vi "AlliGator All ROIs Decay Fit.vi"(8 "error in (no error)":errorcluster, 10 "Lifetime Graph":refnum<vi>, 11 "AlliGator Internal Variables DVR":refnum<data-value>) -> (0 "error out":errorcluster, 1 "Message":string, 3 "AlliGator Internal Variables DVR":refnum<data-value>)   [LabVIEW 2021, in "AlliGator Decay Analysis.lvlib" / "AlliGator Decay Fit.lvlib"]
doc: "Fits all ROI decays with the selected model, using a common IRF for all ROIs."
uses:
  AlliGator Decay Fit.lvlib
  AlliGator Variables List.ctl
  AlliGator Globals, Variables & Constants.lvlib
  Image/Named ROI Description.ctl
  Image/Image.lvlib
  AlliGator Decay Processing.lvlib
  AlliGator Source Image.lvlib
  Strings/Strings.lvlib
  Time/Time.lvlib
  Graphs/XY Graph/XY Graph Add-Ons.lvlib
  AlliGator Settings.lvlib
  AlliGator Settings List.ctl
  Graphs/XY Graph/XY Graph Selected Plot Info+Flag.ctl
  <vilib>/Utility/miscctls.llb/LVPoint32TypeDef.ctl
  Graphs/XY Graph/XY Graph Refnum.ctl
  AlliGator Decay Preprocessing.lvlib
  AlliGator Abort.vi
  Fits/Fits.lvlib
  Variant/Variant to Data/Variant to Data.lvlib
  Variant/Variant to Data/Variant to Boolean.vi
  <vilib>/ErrorRing/Error Ring.xnode
  Notebook/Notebook.lvlib
  Rich Text Box/Rich Text Box.lvlib
  <vilib>/vision/Image Controls.llb/IMAQ Image.ctl
  <vilib>/Utility/error.llb/Error Cluster From Error Code.vi
  GUI/GUI.lvlib
  Fits/IRF(X)PSED/Decay Fit Parameters & Derived Quantities List.ctl
  Utilities/Utilities.lvlib
  Error/Error.lvlib
  Variant/Variant to Data/Variant to U16.vi
  AlliGator Decay Fit Parameter Map.lvlib
  Phasor/Phasor Reference Series.ctl
  Phasor/Phasor.lvlib
  Phasor/Phasor (g, s).ctl
  Phasor/Calibration Phasor (m, phi).ctl
  AlliGator Data Series Type.ctl
  AlliGator Files.lvlib
  AlliGator Internal Variables v2.ctl
  AlliGator Internal Variables.lvlib
  AlliGator Decay Metadata v3.ctl
  AlliGator Phasor Graph.lvlib
  AlliGator Raw Phasor Plot Data v4.ctl
  AlliGator Baseline Subtraction Method.ctl
  AlliGator Decay Background Subtraction Info.ctl
  Graphs/XY Graph/XY Graph Plot Shift Method.ctl
  Graphs/XY Graph/XY Graph Plot Shift Parameters.ctl
  AlliGator Decay Extrapolation Parameters.ctl
  AlliGator FLI Dataset Type.ctl
  Phasor/Phasor Harmonic Data.ctl
  AlliGator Phasor Multi-Harmonic Data.ctl
  AlliGator Phasor Plot.lvlib
  AlliGator Displayed Image.ctl
  Fits/IRF(X)PSED/Decay Fit Parameters In List.ctl
  AlliGator Decay Fit Parameter Constraints 2.ctl
  Fits/Decay Convolution/Decay Model.ctl
  Fits/Residual Type.ctl
  Fits/Fit Calculation Method.ctl
  Fits/Non-linear Fitting Algorithm.ctl
  AlliGator Decay Fit Options & Parameters v2.ctl
  Fits/IRF(X)PSED/Fit Weights Type.ctl
  AlliGator Gate Image Set.ctl
  AlliGator Gate Arithmetic.ctl
  AlliGator Dataset Channel.ctl
  AlliGator Dual-Channel Datasets.lvlib
  AlliGator Decay Preprocessing Parameters.ctl
  Phasor/Phasor Standard Deviation Options.ctl
  Phasor/Phasor Calibration Map v2.ctl
  Fits/Non-linear Fitting Method v2.ctl
  Fits/IRF(X)PSED/Decay Fit Options v2.ctl
  Fits/IRF(X)PSED/MLE Baseline Offset Type.ctl
  AlliGator Parameter Maps Data.ctl
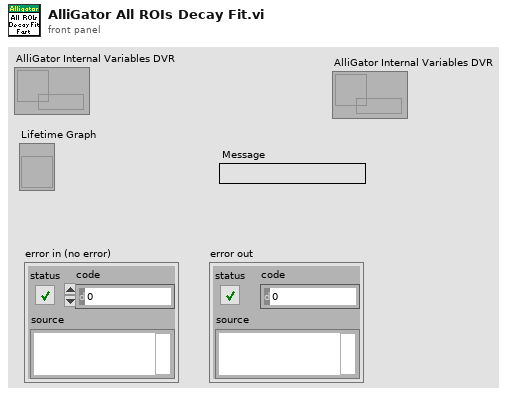
[diagram p1: front panel]
types:
  T1 = typedef "AlliGator Decay Analysis.lvlib/AlliGator Decay Fit.lvlib/AlliGator Decay Fit Output Options.ctl" = cluster{"Fit Model":T2, "Decay Fit Parameter Array":T3[]}
  T2 = typedef "Fits.lvlib/Decay Model.ctl" = enum16{"1-Exponential", "2-Exponentials"}
  T3 = typedef "Fits.lvlib/Decay Fit Parameters & Derived Quantities List.ctl" = enum16{"Offset", "Baseline", "A_1", "tau_1", "A_2", "tau_2", "<tau>_a", "f1_a", "f2_a", "<tau>_i", "f1_i", "f2_i", "-", "R^2", "Chi^2"}
  T4 = typedef "AlliGator Globals, Variables & Constants.lvlib/AlliGator Variables List.ctl" = enum16{"---- GUI ----", "GUI:Initialization Status", "GUI:State Indicators Refnum", "GUI:Original AlliGator Menu Items", "GUI:Current Action Loop State", "GUI:Script in progress", "GUI:Playback", "GUI:Loop Playback", "GUI:Search ROI Used", "GUI:Search ROI", "Decay Graph Max Legend Size", "Intensity Graph Max Legend Size", "Decay Statistics Graph Max Legend Size", "Phasor Graph Max Legend Size", "Phasor Ratio Graph Max Legend Size", "Lifetime Graph Max Legend Size", "---- Files ----", "Files:Export Dataset Frames as Individual Files", "Files:Show Batch Export Help Balloons", "Files:Frames in Dataset", "Files:ptu File Frame Start Indices", "Files:Current Frame in Dataset", "Files:Current Frame Timestamp", "Files:Dataset Loaded", "Files:Dataset Metadata", "Files:Dataset Channel", "Files:Dataset Data Description", "Files:Background Dataset Metadata", "Files:Background Dataset Channel", "Files:Background Dataset Data Description", "Files:Background File Subtraction", "Files:Background File Path", "Files:Background File Pile-up Correction", "Files:Background File Pixel Well Capacity", "Files:Background File Scaling Factor", "Files:Current Dataset Load Settings", "Files:Dataset Path", "Files:ICCD-specific Information", "Files:Macrotime Gate Separation", "------ Python Plugins ------", "Python Plugins:Information", "Python Plugins:Python Session", "Python Plugins:Valid Python Session?", "---- Source Image ----", "Source Image:ROIs", "Source Image:Current ROI", "Source Image:ROI Event Refnum", "X_Source Image Display Range", "X_Source Image Palette Information", "X_Type of Displayed Image", "X_Time Gate Slider", "Source Image:Palette List", "Source Image:Scale", "Source Image:ROI Overlay Color", "Source Image:Overlay to Erase", "Source Image:Is Displayed Image Accumulated", "Source Image:White Light Image Modified", "Source Image:Mask Image Modified", "---- Image Profile Window ----", "Image Profile:Overlay ROI in Source Image", "Image Profile:Window Event Refnum", "Image Profile:IntensityType", "Image Profile:Intensity Average Type", "Image Profile:Intensity-weighted SDV", "Image Profile:Box Profile Type", "Image Profile:Window Open", "Image Profile:Plotted Fit Parameter", "------ Phasor Graph -------", "Phasor Graph:Show Line", "---- Phasor Plot ---", "Phasor Plot:Parameters Changed", "Phasor Plot:FLI Dataset Modified since last Calculation", "Phasor Harmonics Data", "Selected Phasor Harmonics", "Phasor Harmonic Manager Event Refnum", "Phasor Plot:ROIs", "Phasor Plot:Current ROI", "Phasor Plot:ROI Event Refnum", "Phasor Plot:Image Reference Points", "Phasor Plot:Computed", "Phasor Plot:Palette Information", "Phasor Plot:Palette List", "Phasor Plot:Phasor Ratio Palette Information", "Phasor Plot:Phasor Ratio Palette List", "Phasor Plot:Image Scale", "Phasor Plot:Image Overlay to Erase", "Phasor Plot:Image Elements to Update", "Phasor Plot:Current Calculation Parameters", "Phasor Plot:Current Calibration Options", "Phasor Plot:Reset Cumulated Phasor Plot", "Phasor Plot:Reference 1", "Phasor Plot:Lifetime Reference 1", "Phasor Plot:Reference 1 Frequency", "Phasor Plot:Reference 2", "Phasor Plot:Lifetime Reference 2", "Phasor Plot:Reference 2 Frequency", "---- Decay Analysis ----", "Number of Selected Decays to Fit", "LS Fit Results", "LAR Fit Results", "BS Fit Results", "Last Decay Max - Min", "Best Fit Parameters", "Best Fit Parameter Names", "Actual Size X", "Actual Size Y", "Binning X", "Binning Y", "Actual # Gates", "Dataset Number", "Gates to...", "Gates Skipped", "Gates to keep", "Gate Step", "Gate Separation", "Reversed Gates", "Pile-up Correction", "Pixel Well Capacity", "Background Subtracted", "Background Subtraction Method", "Background Definition Range", "Background File (deprecated)", "Number of Dataset Accumulated", "Array of Accumulated Dataset Paths", "Do Averaged Datasets", "Destination File Path", "Process Plot Target", "Use 1/D as Phasor Frequency", "---- Decay Fit Parameter Map -----", "Decay Fit Parameter Map:Palette Information", "Decay Fit Parameter Map:Palette List", "------- Local Decay Window ---------", "Local Decay Graph Window:Event Refnum", "Local Decay Graph Window:Use normalized IRF for convolution", "----- Miscellaneous ----", "Misc:Skippable Dialog Windows Status"}
  T5 = typedef "IMAQ Image.ctl" = refnum<image>
  T6 = typedef "AlliGator Settings.lvlib/AlliGator Settings List.ctl" = enum16{"GUI:Visible Settings Tab", "GUI:Last Run Version", "Source Image:Use Image Histogram for Contrast", "Source Image:Low Count Pixels Rejection Options", "Source Image:High Count Pixels Rejection Options", "Source Image:Use Image Brightness", "Source Image:Blend Overlay with Image Background", "Source Image:Use Fixed ROI Diameter", "Source Image:ROI Diameter", "Source Image:ROI Center Color", "Source Image:Peak Threshold", "Source Image:Intensity Threshold", "Source Image:Image Binning Options", "Source Image:Image Smoothing Options", "Source Image:Image Histogram Active", "Source Image:Invert Binary Mask", "Source Image:Hot Pixel Removal", "Source Image:Overlay Analyzed ROI Center", "Source Image:Auto-Adjust Contrast", "Source Image:Histogram Lower Percentile", "Source Image:Histogram Upper Percentile", "Source Image:Save Source Image", "Source Image:Scale Bar Options", "Source Image:Image Resolution (Pixel Size)", "Source Image:Flatfield Correction", "Source Image:Show Dead Left Columns Correction", "Source Image:Dead Left Columns Correction", "Source Image:Image Pre-Processing Operations Order", "Data Information:Gate Width", "Data Information:Nanotime Gate Separation", "Data Information:Macrotime Gate Separation", "Data Information:Gate Step", "Data Information:# Gates", "Data Information:Gate Image Exposure", "Data Information:Gate Image Integration", "Data Information:Gates to Skip", "Data Information:Gates to Keep", "Data Information:Define Gates to", "Data Information:Channel Name", "Data Information:Available Channel Names", "Data Information:Channel Arithmetic", "Data Information:Background File Subtraction", "Data Information:Background File", "Data Information:Background Scaling Factor", "Data Information:Background Pile-up Correction", "Data Information:Background Pixel Well Capacity", "Data Information:Laser Period", "Data Information:SYNC Period", "Data Information:Pile-up Correction", "Data Information:Pixel Well Capacity", "Data Information:Dataset Scaling Factor", "Fluorescence Decay_Decay Pre-Processing:Reverse Gates", "Fluorescence Decay_Decay Pre-Processing:Verbose Decay Pre-Processing", "Fluorescence Decay_Decay Pre-Processing:Use Decay Pre-Processing", "Fluorescence Decay_Decay Pre-Processing:Background Subtraction", "Fluorescence Decay_Decay Pre-Processing:Background Definition Range", "Fluorescence Decay_Decay Pre-Processing:Baseline Subtraction Method", "Fluorescence Decay_Decay Pre-Processing:Decay Pre-Processing Operations Order", "Fluorescence Decay_Decay Pre-Processing:Smoothing Parameter", "Fluorescence Decay_Decay Pre-Processing:Shift Decay", "Fluorescence Decay_Decay Pre-Processing:Decay Shift Parameters", "Fluorescence Decay_Decay Pre-Processing:Fold Decay", "Fluorescence Decay_Decay Pre-Processing:# Folds", "Fluorescence Decay_Decay Pre-Processing:1-Normalize Decay", "Fluorescence Decay_Decay Pre-Processing:[0-1]-Normalize Decay", "Fluorescence Decay_Decay Pre-Processing:Smoothen Decay", "Fluorescence Decay_Decay Pre-Processing:Extrapolate Decay", "Fluorescence Decay_Decay Pre-Processing:Use Periodicity", "Fluorescence Decay_Decay Pre-Processing:Use Cursors", "Fluorescence Decay_Decay Pre-Processing:Tail Fraction", "Fluorescence Decay_Decay Pre-Processing:Head Fraction", "Fluorescence Decay_Decay Pre-Processing:Additional Points", "Fluorescence Decay_Decay Pre-Processing:Straighten Decay", "Fluorescence Decay_Decay Pre-Processing:Constant Background", "Fluorescence Decay_Decay Pre-Processing:Pixel-Normalize Decay", "Fluorescence Decay_Advanced Analysis:Extract IRF instead of Decay", "Fluorescence Decay_Advanced Analysis:IRF Extraction Options", "Fluorescence Decay_Advanced Analysis:IRF Optimization Options", "Fluorescence Decay_Advanced Analysis:Square Pulse Options", "Fluorescence Decay_Advanced Analysis:IRF Order", "Fluorescence Decay_Advanced Analysis:IRF Time Constants", "Fluorescence Decay_Advanced Analysis:Wavelet Analysis Options", "Fluorescence Decay_Advanced Analysis:Average Lifetime Options", "Fluorescence Decay_Fit Options:Fit Options", "Fluorescence Decay_Fit Options:Use Legacy Fitting Approach", "Fluorescence Decay_Fit Options:Use Data Information Laser Period", "Fluorescence Decay_Fit Parameters:Displayed Fit Parameters", "Fluorescence Decay_Fit Parameters:Fit Parameter Constraints", "Fluorescence Decay_Fit Parameters:Export Tabulated Results", "Fluorescence Decay_Fit Parameters:MLE Baseline Offset Type", "Fluorescence Decay_Fit Parameters:MLE Baseline Offset", "Fluorescence Decay_Fit Parameters:Guess Parameter Names", "Fluorescence Decay_Fit Parameters:Guess Parameter Values", "Fluorescence Decay_Fit Parameters:Guess Parameters Options", "Fluorescence Decay_Styles:Show Last Decay Only", "Fluorescence Decay_Styles:Decay Graph Color Array", "Fluorescence Decay:Decay Graph Active", "Fluorescence Decay Statistics:Min Peak Value", "Fluorescence Decay Statistics:Reject Low Decay Peak Pixels", "Fluorescence Decay Statistics:Reject High Decay Peak Pixels", "Fluorescence Decay Statistics:Max Peak Value", "Time Traces:Use File Timestamp", "Time Traces:Time Step", "Time Traces:Use Intensity Correction File", "Time Traces:Intensity Correction File", "Phasor Plot:Phasor Plot Smoothing Options", "Phasor Plot:Phasor Plot Size", "Phasor Plot:Phasor Plot Graphics Options", "Phasor Plot:Cumulative Phasor Plot", "Phasor Plot:Use Phasor Brightness", "Phasor Plot:Blend Overlay with Phasor Background", "Phasor Plot:Save Phasor Plot", "Phasor Plot:Show References", "Phasor Plot:Phasor Ratio Decay Range", "Phasor Plot:Exponential Fading", "Phasor Plot:Phasor Ratio Reference Colors", "Phasor Plot:Reference Radius", "Phasor Plot:Show Color Map Vertices", "Phasor Plot:Phasor Plot Active", "Phasor Plot:Phasor Ratio Color Map Type", "Phasor Plot:Phasor Ratio Color Map", "Phasor Plot:Phasor Ratio Display Range", "Phasor Plot:Selected Image ROI(s)", "Phasor Plot:All Image ROIs", "Phasor Plot:Selected Phasor Plot ROI(s)", "Phasor Plot:All Phasor Plot ROIs", "Phasor Plot:Phasor Ratio Color-Coded Quantity", "Phasor Plot:Store Phasor Harmonics", "Phasor Plot:Draw Reference Segment", "Phasor Plot:User-Defined Quantity", "Phasor Graph:Phasor Frequency", "Phasor Graph:Phasor Ratio Type", "Phasor Graph:Pixel-level Phasor Computation", "Phasor Graph:Save Phasor Graph", "Phasor Graph:Phasor Graph Active", "Phasor Graph:Phasor SDV Options", "Phasor Calibration:Use Backup Calibration if needed", "Phasor Graph:Define Shortest Lifetime as", "Phasor Calibration:Backup Calibration Type", "Phasor Calibration:Calibration Type", "Phasor Calibration:Calibration Lifetime", "Phasor Calibration:Calibration Map Algorithm", "Single-Exponential Phasor Locus (SEPL):Gate Parameters", "Single-Exponential Phasor Locus (SEPL):User-defined Gate", "Single-Exponential Phasor Locus (SEPL):User-defined IRF", "Single-Exponential Phasor Locus (SEPL):Phasor Parameters", "Single-Exponential Phasor Locus (SEPL):Decay & IRF Parameters", "Single-Exponential Phasor Locus (SEPL):Display Parameters", "Lifetime Analysis:Decay Analysis Parameters", "Lifetime Analysis:Lifetime Map Active", "Plugins:Python Settings", "Miscellaneous:Verbose Mode", "Miscellaneous:Beep after Script", "Miscellaneous:Saved Image File Format", "Miscellaneous:Exported Gate Image Settings", "Miscellaneous:Include Loading in Timing", "Miscellaneous:Verbose Settings Mode", "Miscellaneous:Histogram Options", "Miscellaneous:Beep on Error", "Miscellaneous:# Logical Processors Used", "Miscellaneous:ROI Description Max Characters", "Miscellaneous:Verbose Error Mode", "Miscellaneous:Transparent Mask Color"}
  T7 = typedef "Image.lvlib/Named ROI Description.ctl" = cluster{"ROI Descriptor":T8, "ROI Name":string, "Overlay Color":u32}
  T8 = typedef "ROI Descriptor" = cluster{"Global Rectangle":i32[], "Contours":cluster{"ID":enum32{"External", "Internal"}, "Type":u32, "Coordinates":i32[]}[]}
  T9 = typedef "XY Graph Add-Ons.lvlib/XY Graph Selected Plot Info+Flag.ctl" = cluster{"Multiplot XY Graph":T10, "Mouse Coordinates":T11, "Plot Index":i32, "Flag":bool}
  T10 = typedef "XY Graph Add-Ons.lvlib/XY Graph Refnum.ctl" = refnum<vi>
  T11 = typedef "LVPoint32TypeDef.ctl" = cluster{"Horizontal":i32, "Vertical":i32}
  T12 = typedef "AlliGator Internal Variables.lvlib/AlliGator Internal Variables v2.ctl" = cluster{"Displayed Image":T5, "White Light Image":T5, "Mask Image":T5, "ROI Mask Image":T5, "Current Dataset Images 1":T13, "Background Dataset Images 1":T13, "Current Dataset Images 2":T13, "Background Dataset Images 2":T13, "Current Dataset Arithmetic Images":T13, "Accumulated Dataset Images 1":T13, "Accumulated Dataset Images 2":T13, "Accumulated Dataset Arithmetic Images":T13, "Phasor Plot Image":T5, "Decay Fit Parameter Map Image":T5, "Single Data Point Path":path, "White Light Image Path":path, "Mask Image Path":path, "Time-Series Folder":path, "[Time-Series Paths]":path[], "Current Dataset":i32, "Single Dataset Type":T14, "Current Folder":string, "AlliGator Data Series Type":T15, "# Datasets":i32, "Dual-Channel Dataset":bool, "Selected Channel Name":string, "Dataset Channel":T16, "Channel Arithmetic":T17, "Dual-Channel Background Dataset":bool, "Background Channel":T16, "Dual-Channel Accumulated Dataset":bool, "Start Time":dbl, "[Time-Series Timestamps]":dbl[], "[Intensity Corrections]":dbl[], "Time Series Script":bool, "Type of Displayed Image":T18, "Gate Image Slide":u16, "# Gates":i32, "ROIs":T7[], "ROI Decay":cluster{"t Array":dbl[], "I Array":dbl[]}, "Valid Decay":bool, "Decay  Metadata":T19, "Reference Decay Plot Name":string, "Reference Decay":cluster{"t Array":dbl[], "I Array":dbl[]}, "Decay Shift Plot":cluster{"Time Stamps":dbl[], "Decay Shifts":dbl[]}, "[Decays Max Values]":sgl[], "[Decays Min Values]":sgl[], "Calibration Phasor":T25, "Calibration Phasor Series":T26, "Phasor Calibration Map":T27, "Calibration Map MD5 Digest":string, "Last Raw Phasor":T28, "Last Calibrated Phasor":T28, "Last Calibrated Phasor SDV":T28, "Phasor Graph:Phasor Plot":cluster{"g Array":dbl[], "s Array":dbl[]}, "Phasor Graph:Phasor SDV Plot":cluster{"g Array":dbl[], "s Array":dbl[]}, "[Phasor Graph:Raw Phasor Plots]":T29[], "Phasor Plot locked to Ref 1":i32, "[Phasor Plot(s) locked to Ref 1]":i32[], "[Phasor Plot(s) locked to Ref 2]":i32[], "[Pixel Phasors]":T28[], "[[Sum Image]]":dbl[][], "[[CSG Phasors]]":csg[][], "[[Valid Pixel?]]":bool[][], "I/m/phi Dataset":cluster{"I/m/phi Dataset?":bool, "Base Frequency":dbl[unit], "Harmonic Orders":u8[]}, "Multi Phasor Plot Data":T31, "Decay Fit Options & Parameters":T33, "Fit Options: Decay Preprocessing Parameters":T43, "Fit Options: Reference Decay":cluster{"t Array":dbl[], "I Array":dbl[]}, "Is Full Image Parameters Map":bool, "Is Single-Pixels Parameters Map":bool, "NLSF Parameters Map X Resolution":i32, "NLSF Parameters Map Y Resolution":i32, "[Single Decay Fit Parameters]":dbl[], "Fit Model":T2, "[[Multiple Decays Fit Parameters]]":dbl[][], "[[Multiple Decays Fit Parameter SDVs]]":dbl[][], "[[IRFs]]":dbl[][], "IRF Array Time Axis":dbl[], "Decay Array Time Axis":dbl[], "[Decay Fit Parameter Names]":T3[], "[[Phasor Ratios]]":dbl[][], "[[Average Lifetimes]]":dbl[][], "Amplitude Weighted Average Lifetime":bool, "[Decay Sum]":dbl[], "Parameter Maps":T44[], "[[User-defined Quantities]]":dbl[][], "User-defined Quantity":string}
  T13 = typedef "AlliGator Internal Variables.lvlib/AlliGator Gate Image Set.ctl" = cluster{"SGL Image Max":T5, "SGL Image Sum":T5, "SGL Gate Images":T5[], "SGL Image Min":T5}
  T14 = typedef "AlliGator Files.lvlib/AlliGator FLI Dataset Type.ctl" = enum16{"HDF5 FLI Dataset", "Gate Image Folder", ".sdt FLI Dataset (Becker & Hickl)", ".ptu FLI Dataset (PicoQuant)", "SS1 FLI Dataset", "SS2 FLI Dataset", "I/m/phi Dataset", ".bin FLI Dataset (PicoQuant Binned)", ".bin FLI Dataset (Piccolo Binned)"}
  T15 = typedef "AlliGator Files.lvlib/AlliGator Data Series Type.ctl" = enum16{"Not a Supported Series", "Gate Images Folder Series", "SwissSPAD 2 Dataset Series", "B&H FLI Dataset Series", "PicoQuant PTU FLI Dataset Series", "PicoQuant BIN FLI Dataset Series", "Piccolo hist BIN FLI Dataset Series", "HDF5 FLI Dataset Series"}
  T16 = typedef "AlliGator Dual-Channel Datasets.lvlib/AlliGator Dataset Channel.ctl" = enum16{"G2", "INT"}
  T17 = typedef "AlliGator Settings.lvlib/AlliGator Gate Arithmetic.ctl" = enum16{"None", "INT-G2", "G2/INT*<INT>", "(1 - G2/INT)*<INT>"}
  T18 = typedef "AlliGator Source Image.lvlib/AlliGator Displayed Image.ctl" = enum16{"Single Gate", "Sum of All Gates", "Max of All Gates", "Min of All Gates", "-", "White Ligth Image", "Mask Image"}
  T19 = typedef "AlliGator Phasor Graph.lvlib/AlliGator Decay Metadata v3.ctl" = cluster{"ROI Descriptor":T8, "ROI Center":cluster{"X":i32, "Y":i32}, "Decay Background Subtraction Info":T20, "Decay Reverted":bool, "Decay Smoothened":bool, "Decay Straightened":bool, "Fitted Tau (Decay Straightening)":dbl, "Decay Shift Parameters":T22, "Decay Shifted":bool, "Decay Extrapolated":bool, "Decay Extrapolation Parameters":T24, "Decay Normalized":bool, "Fold Decay":bool, "# Folds":u32}
  T20 = typedef "AlliGator Decay Analysis.lvlib/AlliGator Decay Preprocessing.lvlib/AlliGator Decay Background Subtraction Info.ctl" = cluster{"Laser Period":dbl[unit], "Gate Duration":dbl[unit], "Baseline Subtraction Method":T21, "Background Definition Range":cluster{"Min Gate":dbl[unit], "Max Gate":dbl[unit]}, "Total Intensity w/o Bkgd Subtraction":dbl, "Bkgd-subtracted Intensity (exp)":dbl, "# Data Points":i32, "Background/Gate":dbl, "Fitted Lifetime":dbl[unit], "Bkgd-subtracted Intensity (theo)":dbl}
  T21 = typedef "AlliGator Decay Analysis.lvlib/AlliGator Decay Preprocessing.lvlib/AlliGator Baseline Subtraction Method.ctl" = enum16{"Mean", "Min", "Square Gated Single-Exponential", "File", "Constant"}
  T22 = typedef "XY Graph Add-Ons.lvlib/XY Graph Plot Shift Parameters.ctl" = cluster{"Type":T23, "Shift":dbl[unit], "Threshold":dbl, "Rotate":bool}
  T23 = typedef "XY Graph Add-Ons.lvlib/XY Graph Plot Shift Method.ctl" = enum16{"Default", "CFD", "Threshold", "Cross-Correlation"}
  T24 = typedef "AlliGator Decay Analysis.lvlib/AlliGator Decay Preprocessing.lvlib/AlliGator Decay Extrapolation Parameters.ctl" = cluster{"Additional Points":u32, "Head Fraction":dbl, "Fitted Tau":dbl, "Use Periodicity":bool, "Use Cursors":bool, "Tail Fraction":dbl}
  T25 = typedef "Phasor.lvlib/Calibration Phasor (m, phi).ctl" = cluster{"m":dbl, "phi":dbl, "Phasor Frequency":dbl[unit], "Reference Lifetime":dbl[unit]}
  T26 = typedef "Phasor.lvlib/Phasor Reference Series.ctl" = cluster{"m Array":dbl[], "phi Array":dbl[], "Phasor Frequency":dbl[unit], "Calibration Lifetime":dbl[unit]}
  T27 = typedef "Phasor.lvlib/Phasor Calibration Map v2.ctl" = cluster{"Phasor Frequency":dbl[unit], "Calibration Lifetime":dbl[unit], "ROI Centers":cluster{"X":i32, "Y":i32}[], "ROI Descriptors":T8[], "Map Resolution X":i32, "Map Resolution Y":i32, "z Array":cdb[]}
  T28 = typedef "Phasor.lvlib/Phasor (g, s).ctl" = cluster{"g":dbl, "s":dbl}
  T29 = typedef "AlliGator Phasor Graph.lvlib/AlliGator Raw Phasor Plot Data v4.ctl" = cluster{"Phasor Plot Name":string, "Raw Phasor Plot":T28[], "Phasor Frequency":dbl[unit], "[Decay Metadata]":T19[], "Raw Phasor Plot SDV":T28[], "Phasor SDV Options":T30, "[Calibration Phasor]":T25[]}
  T30 = typedef "Phasor.lvlib/Phasor Standard Deviation Options.ctl" = cluster{"Compute Estimated SDV":bool, "# Replicas":u32, "Use Estimated Average Phasor":bool}
  T31 = typedef "AlliGator Phasor Plot.lvlib/AlliGator Phasor Multi-Harmonic Data.ctl" = cluster{"Base Frequency":dbl[unit], "# Harmonics":u8, "Harmonic Orders":u8[], "Phasor Plot Settings Checksum":u64, "Phasor Harmonic Data Array":T32[]}
  T32 = typedef "Phasor.lvlib/Phasor Harmonic Data.ctl" = cluster{"Phasor Harmonic Name":string, "Phasor Plot Settings Checksum":u64, "Phasor Frequency":dbl[unit], "Base Frequency":dbl[unit], "Harmonic Order":u8, "Phasor Plot Parameters":string, "Phasor Array [[CSG]]":csg[][], "Dataset File Path":path}
  T33 = typedef "AlliGator Decay Fit Parameter Map.lvlib/AlliGator Decay Fit Options & Parameters v2.ctl" = cluster{"SYNC Period":dbl[unit], "Fit Options":T34, "Fit Parameter Constraints":T40[], "MLE Baseline Offset":dbl, "MLE Baseline Offset Type":T42}
  T34 = typedef "Fits.lvlib/Decay Fit Options v2.ctl" = cluster{"Show Fit Residuals":bool, "Fit Model":T2, "Residual Type":T35, "Max Decay Percentile":dbl, "Min Decay Percentile":dbl, "Show Full Decay":bool, "Weights":T36, "Fitting Method":T37, "Compute Parameter Uncertainties":bool, "Periodic Boundaries":bool, "Model Calculation":T38, "Period":dbl[unit], "Termination Criteria":cluster{"Max Iterations":i32, "Max Function Calls":i32, "Max Time":dbl[unit], "Function Tolerance":dbl, "Parameter Tolerance":dbl, "Gradient Tolerance":dbl, "Min Lambda":dbl, "Max Lambda":dbl, "Initial Tick Count":u32}, "Offset Resolution":dbl[unit], "Use Local IRF":bool, "Fitting Algorithm":T39}
  T35 = typedef "Fits.lvlib/Residual Type.ctl" = enum16{"Standard", "Normalized", "Reduced"}
  T36 = typedef "Fits.lvlib/Fit Weights Type.ctl" = enum16{"Unweighted", "1/Variance", "Best of All"}
  T37 = typedef "Fits.lvlib/Non-linear Fitting Method v2.ctl" = enum16{"Least Square", "Least Absolute Residual", "Bisquare", "MLE", "-", "Best of All"}
  T38 = typedef "Fits.lvlib/Fit Calculation Method.ctl" = enum16{"Simulation", "Convolution", "Integration"}
  T39 = typedef "Fits.lvlib/Non-linear Fitting Algorithm.ctl" = enum16{"Levenberg-Marquardt", "Trust-Region Dogleg"}
  T40 = typedef "AlliGator Decay Analysis.lvlib/AlliGator Decay Fit.lvlib/AlliGator Decay Fit Parameter Constraints 2.ctl" = cluster{"Fit Parameter":T41, "Min Value":dbl, "Max Value":dbl, "Global":bool, "Used":bool}
  T41 = typedef "Fits.lvlib/Decay Fit Parameters In List.ctl" = enum16{"Offset", "Baseline", "A_1", "tau_1", "A_2", "tau_2"}
  T42 = typedef "Fits.lvlib/MLE Baseline Offset Type.ctl" = enum32{"Absolute", "Percentage"}
  T43 = typedef "AlliGator Decay Analysis.lvlib/AlliGator Decay Preprocessing.lvlib/AlliGator Decay Preprocessing Parameters.ctl" = cluster{"Background Subtraction":bool, "Straighten Decay":bool, "Reverse Gates":bool, "1-Normalized Decay":bool, "Smoothen Decay":bool, "Smoothing Parameter":dbl, "Shift Decay":bool, "Decay Shift Parameters":T22, "Extrapolate Decay":bool, "Additional Points":u32, "Head Fraction":dbl, "Pixel-Normalize Decay":bool, "Use Periodicity":bool, "Use Cursors":bool, "Tail Fraction":dbl, "Use Decay Pre-Processing":bool, "Fold Decay":bool, "# Folds":u32, "[0-1]-Normalized Decay":bool}
  T44 = typedef "AlliGator Parameter Maps Data.ctl" = cluster{"Map Set Name":string, "[Parameter Names]":string[], "[[Parameters]]":dbl[][], "[[Parameter SDVs]]":dbl[][], "Decay Array Time Axis":dbl[], "[[IRFs]]":dbl[][], "IRF Array Time Axis":dbl[]}
  T45 = typedef "AlliGator Settings.lvlib/AlliGator Pixel Counts Constraints.ctl" = cluster{"High Count Pixels Rejection Options":T46, "Low Count Pixels Rejection Options":T47}
  T46 = typedef "AlliGator Settings.lvlib/AlliGator High Count Pixels Rejection Options.ctl" = cluster{"Background High Threshold Factor":dbl, "Fixed High Background Threshold":dbl, "Reject High Count Pixels":bool, "High Percentile":dbl}
  T47 = typedef "AlliGator Settings.lvlib/AlliGator Low Count Pixels Rejection Options.ctl" = cluster{"Background Low Threshold Factor":dbl, "Fixed Low Background Threshold":dbl, "Reject Low Count Pixels":bool, "Low Percentile":dbl}
  T48 = cluster{"Decay Peak Constraint":bool, "Min":dbl, "Max":dbl}
  T49 = typedef "Rich Text Box.lvlib/Text Formatting.ctl" = cluster{"Font":string, "Text Color":T50, "Text Background Color":T50, "Text Style":enum16{"Regular", "Bold", "Italic", "Underline", "Strikeout"}, "Font Size (Points)":dbl, "Text Alignment":i32}
  T50 = typedef "Rich Text Box.lvlib/Text Colors.ctl" = enum16{"Unchanged", "Black", "Blue", "Brown", "Gray", "Green", "Orange", "Pink", "Red", "White"}
  T51 = cluster{"t Axis":dbl[], "ROI Intensity Array":dbl[]}
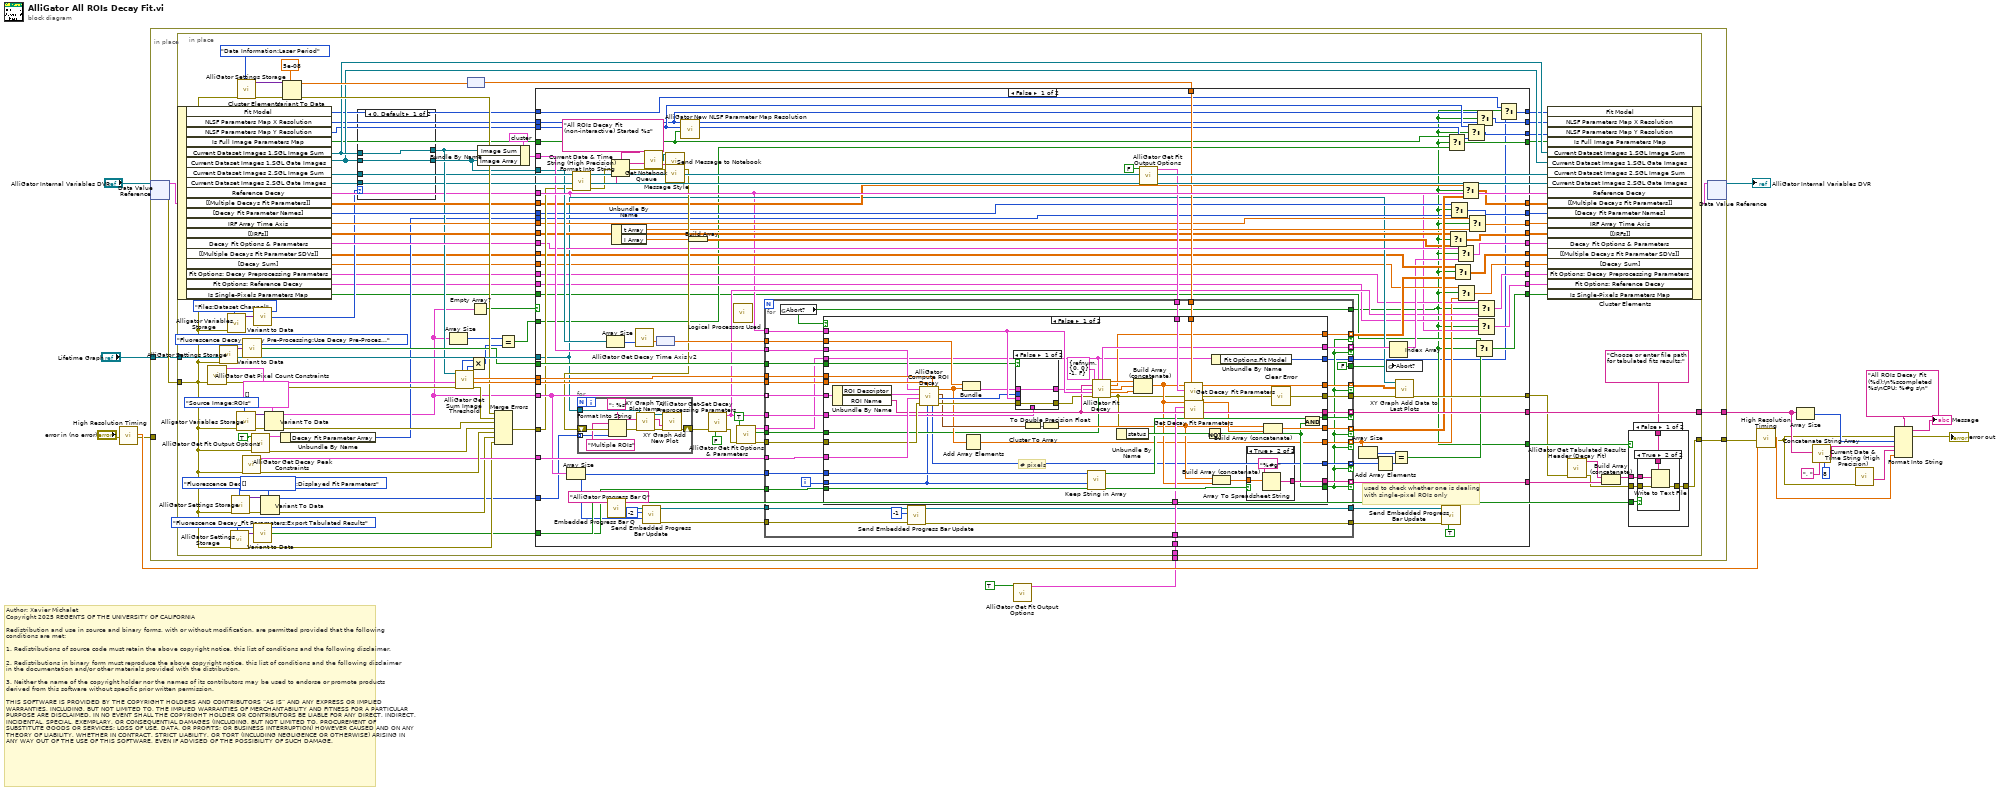
[diagram p0: block diagram]
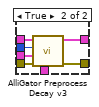
[diagram p3: hidden frame]
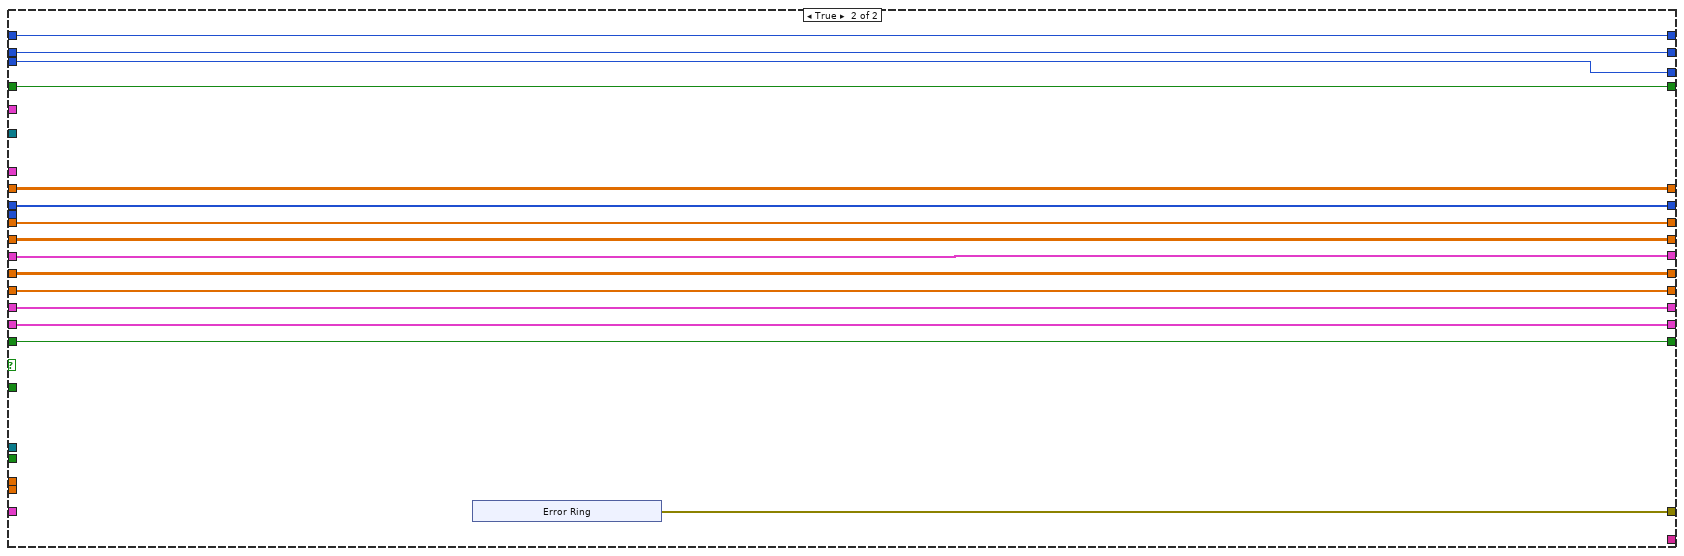
[diagram p6: hidden frame]
diagram:
  # "Author: Xavier Michalet\nCopyright 2025 REGENTS OF THE UNIVERSITY OF CALIFORNIA\n\nRedistribution and use in source and binary forms, with or without modification, are permitted provided that the following conditions are met:\n\n1. Redistributions of source code must retain the above copyright notice, this list of conditions and the following disclaimer.\n\n2. Redistributions in binary form must reproduce the above copyright notice, this list of conditions and the following disclaimer in the documentation and/or other materials provided with the distribution.\n\n3. Neither the name of the copyright holder nor the names of its contributors may be used to endorse or promote products derived from this software without specific prior written permission.\n\nTHIS SOFTWARE IS PROVIDED BY THE COPYRIGHT HOLDERS AND CONTRIBUTORS “AS IS” AND ANY EXPRESS OR IMPLIED WARRANTIES, INCLUDING, BUT NOT LIMITED TO, THE IMPLIED WARRANTIES OF MERCHANTABILITY AND FITNESS FOR A PARTICULAR PURPOSE ARE DISCLAIMED. IN NO EVENT SHALL THE COPYRIGHT HOLDER OR CONTRIBUTORS BE LIABLE FOR ANY DIRECT, INDIRECT, INCIDENTAL, SPECIAL, EXEMPLARY, OR CONSEQUENTIAL DAMAGES (INCLUDING, BUT NOT LIMITED TO, PROCUREMENT OF SUBSTITUTE GOODS OR SERVICES; LOSS OF USE, DATA, OR PROFITS; OR BUSINESS INTERRUPTION) HOWEVER CAUSED AND ON ANY THEORY OF LIABILITY, WHETHER IN CONTRACT, STRICT LIABILITY, OR TORT (INCLUDING NEGLIGENCE OR OTHERWISE) ARISING IN ANY WAY OUT OF THE USE OF THIS SOFTWARE, EVEN IF ADVISED OF THE POSSIBILITY OF SUCH DAMAGE."
  n1 = call "High Resolution Timing.vi"("Error In"="error in (no error)") -> ("elapsed (relative) seconds"=w14:dbl, "Error Out"=w9:errorcluster)  [unwired: 16 in, 1 out]
  n2 = call "AlliGator Get Fit Output Options.vi"("All Parameters?"=TRUE) -> ("Decay Fit Output Options"=w5:T1)  [unwired: 8 in, 2 out]
  n3 = in-place {
    in-place-border: [w25] -> w7
    in-place-border: [w24] -> w11
    in-place-border: w9 -> [_]
    in-place-border: "Lifetime Graph" -> [w22]
    in-place-border: w5 -> [w21]
    n4 = in-place-dvr #1("AlliGator Internal Variables DVR") -> (w27:T12, w23:errorcluster)
    n5 = in-place {
      in-place-border: w23 -> [w55]
      in-place-border: [w95] -> w25
      in-place-border: [w111] -> w24
      in-place-border: w22 -> [w103]
      in-place-border: w21 -> [w91]
      w106 = T3[] [] items=["Offset", "Baseline", "A_1", "tau_1", "A_2", "tau_2", "<tau>_a", "f1_a", "f2_a", "<tau>_i", "f1_i", "f2_i", "-", "R^2", "Chi^2"] ("Array")
      n6 = in-place-cluster #2(w27) -> ("Fit Model"=w29:T2, "NLSF Parameters Map X Resolution"=w35:i32, "NLSF Parameters Map Y Resolution"=w32:i32, "Is Full Image Parameters Map"=w43:bool, "Current Dataset Images 1.SGL Image Sum"=w49:T5, "Current Dataset Images 1.SGL Gate Images"=w48:T5[], "Current Dataset Images 2.SGL Image Sum"=w67:T5, "Current Dataset Images 2.SGL Gate Images"=w66:T5[], "Reference Decay"=w64:cluster{"t Array":dbl[], "I Array":dbl[]}, "[[Multiple Decays Fit Parameters]]"=w80:dbl[][], "[Decay Fit Parameter Names]"=w77:T3[], "IRF Array Time Axis"=w75:dbl[], "[[IRFs]]"=w74:dbl[][], "Decay Fit Options & Parameters"=w71:T33, "[[Multiple Decays Fit Parameter SDVs]]"=w52:dbl[][], "[Decay Sum]"=w51:dbl[], "Fit Options: Decay Preprocessing Parameters"=w47:T43, "Fit Options: Reference Decay"=w45:cluster{"t Array":dbl[], "I Array":dbl[]}, "Is Single-Pixels Parameters Map"=w31:bool)
      n7 = call "AlliGator Get Pixel Count Constraints.vi"("error in (no error)"=w55) -> ("error out"=w118:errorcluster, "Pixel Count Constraints"=w119:T45)  [unwired: 9 in]
      n8 = call "AlliGator Settings Storage.vi"("AlliGator Settings List"=AlliGator_Settings_List."Fluorescence Decay_Decay Pre-Processing:Use Decay Pre-Processing", "Error In"=w55) -> ("Variant Data out"=w83:variant)  [unwired: 8 in, 1 out]
      n9 = call "Alligator Variables Storage.vi"("AlliGator Variable"=AlliGator_Variables_List."Files:Dataset Channel" ("Alligator Variable"), "Error In"=w55) -> ("Data out"=w56:variant)  [unwired: 7 in, 2 out]
      n10 = call "AlliGator Settings Storage.vi"("AlliGator Settings List"=AlliGator_Settings_List."Fluorescence Decay_Fit Parameters:Export Tabulated Results", "Error In"=w55) -> ("Error Out"=w100:errorcluster, "Variant Data out"=w101:variant)  [unwired: 8 in]
      n11 = call "AlliGator Settings Storage.vi"("AlliGator Settings List"=AlliGator_Settings_List."Fluorescence Decay_Fit Parameters:Displayed Fit Parameters", "Error In"=w55) -> ("Error Out"=w108:errorcluster, "Variant Data out"=w107:variant)  [unwired: 8 in]
      n12 = call "Alligator Variables Storage.vi"("AlliGator Variable"=AlliGator_Variables_List."Source Image:ROIs" ("Alligator Variable"), "Error In"=w55) -> ("Error Out"=w121:errorcluster, "Data out"=w122:variant)  [unwired: 7 in, 1 out]
      n13 = call "AlliGator Settings Storage.vi"("AlliGator Settings List"=AlliGator_Settings_List."Data Information:Laser Period", "Error In"=w55) -> ("Error Out"=w89:errorcluster, "Variant Data out"=w90:variant)  [unwired: 8 in]
      n14 = call "AlliGator Get Decay Peak Constraints.vi"("error in (no error)"=w55) -> ("Error Out"=w114:errorcluster, "Decay Peak Constraints"=w113:T48)  [unwired: 9 in]
      n15 = call-poly "Variant to Data.vi"("Variant"=w83) -> ("Value"=w81:bool)  [unwired: 8 in]
      n16 = call "AlliGator Get Fit Output Options.vi"("Error In"=w55, "All Parameters?"=TRUE) -> ("Error Out"=w58:errorcluster, "Decay Fit Output Options"=w61:T1)  [unwired: 7 in, 1 out]
      n17 = call-poly "Variant to Data.vi"("Variant"=w56) -> ("U16 Value"=w54:u16)  [unwired: 8 in]
      n18 = call-poly "Variant to Data.vi"("Variant"=w101) -> ("Value"=w93:bool)  [unwired: 8 in]
      n19 = Variant To Data(error in=w108, type=w106, Variant=w107) -> (data=w62:T3[], error out=w104:errorcluster)
      n20 = Variant To Data(error in=w121, type=T7[] [] ("Stored ROIs in"), Variant=w122) -> (data=w41:T7[], error out=w117:errorcluster)
      n21 = Unbundle By Name(w61) -> ("Decay Fit Parameter Array"=w59:T3[])
      n22 = Variant To Data(error in=w89, type=dbl[unit] 5e-08 ("Laser Period"), Variant=w90) -> (data=w88:dbl[unit], error out=w84:errorcluster)
      n23 = case shown="0, Default" w54 {
        tunnel: [w125 w127] -> w68
        tunnel: w67 -> [_ w127]
        tunnel: w66 -> [_ w126]
        tunnel: [w124 w126] -> w69
        tunnel: w49 -> [w125 _]
        tunnel: w48 -> [w124 _]
        frame 0, Default {
        }
        frame 1 {
        }
      }
      n24 = Array Size(array=w41) -> (size(s)=w38:i32)
      n25 = call "AlliGator Get Sum Image Threshold.vi"("error in (no error)"=w118, "Pixel Counts Constraints"=w119, "Image in"=w68) -> ("error out"=w110:errorcluster, "Pixel Threshold Low"=w115:sgl, "Pixel Threshold High"=w116:sgl, "Y Resolution"=w40:i32, "X Resolution"=w39:i32)  [unwired: 2 in, 2 out]
      n26 = node(w88) -> (w85:dbl)
      n27 = Multiply(x=w39, y=w40) -> (x*y=w37:i32)
      n28 = Empty Array?(array=w41) -> (empty?=w63:bool)
      n29 = Bundle By Name(cluster=cluster{"Image Sum":T5, "Image Array":T5[]} {"Image Sum"=refnum, "Image Array"=[]} ("Images"), "Image Sum"=w68, "Image Array"=w69) -> (w112:cluster{"Image Sum":T5, "Image Array":T5[]})
      n30 = Merge Errors(w84, w110, w117, w58, w114, w104, w100) -> (w109:errorcluster)
      n31 = Equal?(x=w38, y=w37) -> (x = y?=w36:bool)
      n32 = case shown="False" w63 {
        tunnel: w116 -> [w223 _]
        tunnel: w115 -> [w222 _]
        tunnel: w113 -> [w221 _]
        tunnel: w112 -> [w220 _]
        tunnel: w69 -> [w219 _]
        tunnel: w64 -> [w154 _]
        tunnel: [w216 _] -> w111
        tunnel: w109 -> [w197 _]
        tunnel: w62 -> [w177 _]
        tunnel: w103 -> [w167 _]
        tunnel: [w214 _] -> w99
        tunnel: [w130 _] -> w96
        tunnel: [w213 w348] -> w79
        tunnel: w93 -> [w212 _]
        tunnel: [w195 w349] -> w92
        tunnel: w41 -> [w211 _]
        tunnel: w91 -> [w210 _]
        tunnel: w85 -> [w207 _]
        tunnel: w81 -> [w206 _]
        tunnel: w80 -> [w194 w349]
        tunnel: w77 -> [w193 w347]
        tunnel: [w192 w347] -> w76
        tunnel: w75 -> [w191 w346]
        tunnel: w74 -> [w190 w345]
        tunnel: [w189 w346] -> w73
        tunnel: [w188 w345] -> w72
        tunnel: w71 -> [w183 w344]
        tunnel: [w182 w344] -> w70
        tunnel: w59 -> [w169 _]
        tunnel: [w163 w343] -> w53
        tunnel: w52 -> [w162 w343]
        tunnel: w51 -> [w161 w342]
        tunnel: [w160 w342] -> w50
        tunnel: w47 -> [w158 w341]
        tunnel: [w157 w341] -> w46
        tunnel: w45 -> [w155 w340]
        tunnel: [w153 w340] -> w44
        tunnel: w43 -> [w143 w339]
        tunnel: [w147 w339] -> w42
        tunnel: w36 -> [w144 _]
        tunnel: w35 -> [w139 w338]
        tunnel: w32 -> [w141 w337]
        tunnel: [w146 w338] -> w34
        tunnel: [w145 w337] -> w33
        tunnel: w31 -> [w134 w336]
        tunnel: [w132 w336] -> w30
        tunnel: w29 -> [w131 w335]
        tunnel: [w128 w335] -> w28
        frame False {
          # "used to check whether one is dealing with single-pixel ROIs only"
          n33 = Array Size(array=w211) -> (size(s)=w174:i32)
          n34 = call "Current Date & Time String (High Precision).vi"("Error In"=w197) -> ("Error Out"=w201:errorcluster, "on <Date> at <Time>"=w180:string)  [unwired: 7 in, 2 out]
          n35 = Array Size(array=w219) -> (size(s)=w218:i32)
          n36 = call "Embedded Progress Bar Q.vi"("Progress Bar Queue Name"="AlliGator Progress Bar Q") -> ("Progress Bar Queue"=w179:refnum<queue>)  [unwired: 6 in]
          n37 = Format Into String(format string="All ROIs Decay Fit (non-interactive) Started %s", error in=w201, w180) -> (resulting string=w202:string, error out=w200:errorcluster)  [unwired: 1 in]
          n38 = Unbundle By Name(w154) -> ("t Array"=w187:dbl[], "I Array"=w186:dbl[])
          n39 = call "AlliGator Get Decay Time Axis v2.vi"("Number of Gates"=w218) -> ("t Array"=w217:dbl[unit][])  [unwired: 14 in]
          n40 = call "Send Embedded Progress Bar Update.vi"("Max Iterations N"=w174, "Current Iteration i (i or -1: standard or || iteration; 0 or -2: first standard or || iteration)"=-2 ("Current Iteration i (i or -1: standard or || iteration; 0 or -2: first standard or || iteration)"), "Progress Bar Queue in"=w179) -> ("Error Out"=w173:errorcluster, "Progress Bar Queue out"=w176:refnum<queue>)  [unwired: 7 in]
          n41 = call "Get Notebook Queue.vi"() -> ("Notebook Queue"=w199:refnum<queue>)  [unwired: 9 in]
          n42 = node(w217) -> (w215:dbl[])
          n43 = call "Message Style.vi"() -> ("Message Formatting"=w204:T49)
          n44 = call "Send Message to Notebook.vi"("Text Formatting"=w204, "Error In"=w200, "Message"=w202, "Notebook Queue"=w199) -> ("Error Out"=w198:errorcluster)  [unwired: 4 in, 1 out]
          n45 = for {
            tunnel: w167 -> [w231]
            shift-right: [w233] -> w205
            shift-left: w198 -> [w229]
            tunnel: w177 -> [w225] mode=indexing
            n46 = Format Into String(format string=": %s", initial string="Multiple ROIs", error in=w229, w225) -> (resulting string=w227:string, error out=w228:errorcluster)
            n47 = call "XY Graph Try Plot Name.vi"("Error In"=w228, "Plot Name in"=w227, "XY Graph Refnum"=w231) -> ("Error Out"=w232:errorcluster, "Plot Name out"=w234:string, "XY Graph Refnum"=w224:T10)  [unwired: 5 in, 1 out]
            n48 = call "XY Graph Add New Plot.vi"("Multiplot XY Graph"=w224, "New Plot Name in"=w234, "error in (no error)"=w232) -> ("error out"=w233:errorcluster)  [unwired: 9 in, 3 out]
          }
          n49 = call "AlliGator New NLSF Parameter Map Resolution.vi"("Is Full Image Parameter Map"=w143, "Old NLSF Parameters Map Y Resolution"=w141, "Old NLSF Parameters Map X Resolution"=w139) -> (2:"New NLSF Parameters Map X Resolution"=w142:i32, 3:"New NLSF Parameters Map X Resolution"=w140:i32)  [unwired: 7 in]
          n50 = Build Array(w186) -> (w185:dbl[][])
          n51 = call "AlliGator Get-Set Decay Preprocessing Parameters.vi"("Get (F)/Set"=FALSE, "Error In"=w205) -> ("Error Out"=w152:errorcluster, "Decay Preprocessing Parameters out"=w156:T43)  [unwired: 8 in]
          n52 = call "Logical Processors Used.vi"() -> ()  [unwired: 6 in, 1 out]
          n53 = call "AlliGator Get Fit Options & Parameters.vi"("error in (no error)"=w152, "Reset Fit Options & Parameters"=TRUE) -> ("error out"=w151:errorcluster, "Use Legacy Fitting Approach"=w150:bool, "Decay Fit Options & Parameters"=w149:T33)  [unwired: 7 in]
          n54 = call "AlliGator Get Fit Output Options.vi"("All Parameters?"=FALSE) -> ("Decay Fit Output Options"=w208:T1)  [unwired: 8 in, 2 out]
          n55 = for {
            tunnel: w211 -> [w271] mode=indexing
            tunnel: w223 -> [w270]
            tunnel: w222 -> [w269]
            tunnel: w220 -> [w268]
            tunnel: w221 -> [w267]
            tunnel: w215 -> [w265]
            tunnel: w154 -> [w264]
            tunnel: [w263] -> w216 mode=indexing if=w257
            tunnel: w151 -> [w266]
            tunnel: [w262] -> w166
            tunnel: [w261] -> w214 mode=indexing if=w236
            tunnel: w212 -> [w260]
            tunnel: [w242] -> w130
            tunnel: [w256] -> w196 mode=indexing if=w236
            tunnel: w174 -> [w259]
            tunnel: w210 -> [w255]
            tunnel: w208 -> [w254]
            tunnel: w207 -> [w253]
            tunnel: w206 -> [w252]
            tunnel: [w251] -> w184 mode=indexing if=w236
            tunnel: w156 -> [w250]
            tunnel: w176 -> [w249]
            tunnel: w173 -> [w248]
            tunnel: [w247] -> w172
            tunnel: [w246] -> w171
            tunnel: [w245] -> w168 mode=indexing if=w236
            tunnel: [FALSE ("Abort?")] -> w165
            tunnel: [w241] -> w138 mode=indexing if=w236
            tunnel: [w240] -> w164 mode=indexing if=w236
            tunnel: w150 -> [w239]
            tunnel: w149 -> [w238]
            tunnel: [w237] -> w136 mode=indexing if=w236
            tunnel: [w235] -> w129
            i -> [w258]
            n56 = global read "AlliGator Abort.vi" "Abort?"() -> (w242:bool)
            n57 = case shown="False" w242 {
              tunnel: w271 -> [w321 _]
              tunnel: w270 -> [w320 _]
              tunnel: w269 -> [w319 _]
              tunnel: w268 -> [w318 _]
              tunnel: w267 -> [w317 _]
              tunnel: w266 -> [w316 w334]
              tunnel: w265 -> [w315 _]
              tunnel: w264 -> [w314 _]
              tunnel: [w313 _] -> w263
              tunnel: [w312 w334] -> w262
              tunnel: [w311 _] -> w261
              tunnel: w260 -> [w310 _]
              tunnel: w259 -> [w309 _]
              tunnel: w258 -> [w272 _]
              tunnel: [w308 _] -> w257
              tunnel: [w307 _] -> w256
              tunnel: w255 -> [w306 _]
              tunnel: w254 -> [w305 _]
              tunnel: w253 -> [w304 _]
              tunnel: w252 -> [w303 _]
              tunnel: [w302 _] -> w251
              tunnel: w250 -> [w301 _]
              tunnel: [w300 _] -> w245
              tunnel: [w299 _] -> w236
              tunnel: [w278 _] -> w241
              tunnel: [w277 _] -> w240
              tunnel: w239 -> [w276 _]
              tunnel: w238 -> [w274 _]
              tunnel: [w275 _] -> w237
              tunnel: [w273 _] -> w235
              frame False {
                # "# pixels"
                n58 = Unbundle By Name(w321) -> ("ROI Descriptor"=w298:T8, "ROI Name"=w313:string)
                n59 = call "AlliGator Compute ROI Decay.vi"("Pixel Threshold High"=w320, "Loop ID"=w272, "Pixel Threshold Low"=w319, "error in (no error)"=w316, "Decay Peak  Constraints"=w317, "ROI Descriptor"=w298, "Images"=w318) -> ("error out"=w297:errorcluster, "# Valid Pixels"=w295:i32, "ROI Center"=w284:cluster{"X":i32, "Y":i32}, "Decay Points"=w279:dbl[], "# Pixels"=w275:i32)
                n60 = Bundle(w315, "Decay Points"=w279) -> (w296:cluster{dbl[], "Decay Points":dbl[]})  [unwired: 1 in]
                n61 = Add Array Elements(numeric array=w279) -> (sum=w278:dbl)
                n62 = case shown="False" w303 {
                  tunnel: w297 -> [w322 w330]
                  tunnel: w296 -> [w323 w329]
                  tunnel: w295 -> [_ w328]
                  tunnel: [w322 w327] -> w281
                  tunnel: w314 -> [_ w326]
                  tunnel: [w323 w325] -> w294
                  tunnel: w301 -> [_ w324]
                  frame False {
                  }
                  frame True {
                    n63 = call "AlliGator Preprocess Decay v3.vi"("Decay Preprocessing Parameters"=w324, "Error In"=w330, "Time-Gated Reference Decay"=w326, "# Pixels"=w328, "Decay (in)"=w329) -> ("Error Out"=w327:errorcluster, "Decay (out)"=w325:T51)  [unwired: 3 in, 2 out]
                  }
                }
                n64 = Cluster To Array(cluster=w284) -> (array=w283:i32[])
                n65 = To Double Precision Float(number=w283) -> (double precision float=w282:dbl[])
                n66 = call "Keep String in Array.vi"("Current Index"=w272, "Number of Elements"=w309) -> ("Keep String"=w287:bool)  [unwired: 9 in]
                n67 = call "AlliGator Fit Decay.vi"("Selected Plot Info + Flag"=T9 {"Multiplot XY Graph"=refnum, "Mouse Coordinates"={"Horizontal"=0, "Vertical"=0}, "Plot Index"=-1, "Flag"=FALSE}, "Decay Fit Options & Parameters"=w274, "Current Decay Name"=w313, "Current Decay"=w294, "Reference Decay"=w314, "error in (no error)"=w281, "Use Legacy Fitting Approach"=w276) -> ("Decay Fit Options & Parameters (out)"=w302:T33, "Best Fit Parameters (All)"=w292:dbl[], "Delta Best Fit Parameters (All)"=w277:dbl[], "R^2"=w291:dbl, "Reduced Chi^2"=w290:dbl, "Error Out"=w280:errorcluster)  [unwired: 3 out]
                n68 = Unbundle By Name(w280) -> ("status"=w289:bool)
                n69 = Build Array (concatenate)(w292, w291, w290) -> (w286:dbl[])
                n70 = call "Get Decay Fit Parameters.vi"("Laser Period"=w304, "Decay Fit Output Options"=w305, "Decay Fit Parameters"=w286) -> ("Displayed Decay Fits Parameters"=w300:dbl[])  [unwired: 7 in, 1 out]
                n71 = call "Get Decay Fit Parameters.vi"("Laser Period"=w304, "Decay Fit Output Options"=w306, "Decay Fit Parameters"=w286) -> ("Displayed Decay Fits Parameters"=w285:dbl[])  [unwired: 7 in, 1 out]
                n72 = Not(x=w289) -> (.not. x?=w299:bool)
                n73 = Unbundle By Name(w274) -> ("Fit Options.Fit Model"=w273:T2)
                n74 = Build Array (concatenate)(w282, w286) -> (w288:dbl[])
                n75 = case shown="True" w310 {
                  tunnel: [_ w333] -> w311
                  tunnel: w288 -> [_ w332]
                  frame False {
                  }
                  frame True {
                    n76 = Array To Spreadsheet String(array=w332, 3:"%#g" ("format string")) -> (spreadsheet string=w333:string)  [unwired: 1 in]
                  }
                }
                n77 = Build Array (concatenate)(w282, w285) -> (w307:dbl[])
                n78 = call "Clear Error.vi"("Error In"=w280) -> ("no Error Out"=w312:errorcluster)  [unwired: 8 in]
                n79 = Compound Arithmetic op=AND(w287, w299) -> (w308:bool)
              }
              frame True {
              }
            }
            n80 = call "Send Embedded Progress Bar Update.vi"("Error In"=w248, "Current Iteration i (i or -1: standard or || iteration; 0 or -2: first standard or || iteration)"=-1 ("Current Iteration i (-1: || iteration, -2: first || iteration)"), "Progress Bar Queue in"=w249) -> ("Error Out"=w246:errorcluster, "Progress Bar Queue out"=w247:refnum<queue>)  [unwired: 7 in]
          }
          n81 = Array Size(array=w138) -> (size(s)=w137:i32)
          n82 = Add Array Elements(numeric array=w136) -> (sum=w135:i32)
          n83 = global write "AlliGator Abort.vi" "Abort?"(w165) -> ()
          n84 = Index Array(array=w184) -> (element=w159:T33)  [unwired: 1 in]
          n85 = Equal?(x=w137, y=w135) -> (x = y?=w133:bool)
          n86 = call "XY Graph Add Data to Last Plots.vi"("error in (no error)"=w166, "Plots Data Array"=w168, "XYGraph in"=w167) -> ("error out"=w213:errorcluster)  [unwired: 8 in]
          n87 = call "Send Embedded Progress Bar Update.vi"("Stop Progress Bar (F)"=TRUE, "Error In"=w171, "Progress Bar Queue in"=w172) -> ()  [unwired: 7 in, 2 out]
          n88 = Select(t=w143, s=w130, f=w144) -> (s? t:f=w147:bool)
          n89 = Select(t=w190, s=w130, f=w185) -> (s? t:f=w188:dbl[][])
          n90 = Select(t=w193, s=w130, f=w169) -> (s? t:f=w192:T3[])
          n91 = Select(t=w162, s=w130, f=w164) -> (s? t:f=w163:dbl[][])
          n92 = Select(t=w183, s=w130, f=w159) -> (s? t:f=w182:T33)
          n93 = Select(t=w161, s=w130, f=w138) -> (s? t:f=w160:dbl[])
          n94 = Select(t=w194, s=w130, f=w196) -> (s? t:f=w195:dbl[][])
          n95 = Select(t=w141, s=w130, f=w142) -> (s? t:f=w145:i32)
          n96 = Select(t=w191, s=w130, f=w187) -> (s? t:f=w189:dbl[])
          n97 = Select(t=w134, s=w130, f=w133) -> (s? t:f=w132:bool)
          n98 = Select(t=w139, s=w130, f=w140) -> (s? t:f=w146:i32)
          n99 = Select(t=w158, s=w130, f=w156) -> (s? t:f=w157:T43)
          n100 = Select(t=w155, s=w130, f=w154) -> (s? t:f=w153:cluster{"t Array":dbl[], "I Array":dbl[]})
          n101 = Select(t=w131, s=w130, f=w129) -> (s? t:f=w128:T2)
        }
        frame True {
          n102 = xnode "Error Ring"() -> ("error out"=w348:errorcluster)
        }
      }
      n103 = in-place-cluster #2("Fit Model"=w28, "NLSF Parameters Map X Resolution"=w34, "NLSF Parameters Map Y Resolution"=w33, "Is Full Image Parameters Map"=w42, "Current Dataset Images 1.SGL Image Sum"=w49, "Current Dataset Images 1.SGL Gate Images"=w48, "Current Dataset Images 2.SGL Image Sum"=w67, "Current Dataset Images 2.SGL Gate Images"=w66, "Reference Decay"=w64, "[[Multiple Decays Fit Parameters]]"=w92, "[Decay Fit Parameter Names]"=w76, "IRF Array Time Axis"=w73, "[[IRFs]]"=w72, "Decay Fit Options & Parameters"=w70, "[[Multiple Decays Fit Parameter SDVs]]"=w53, "[Decay Sum]"=w50, "Fit Options: Decay Preprocessing Parameters"=w46, "Fit Options: Reference Decay"=w44, "Is Single-Pixels Parameters Map"=w30) -> (w26:T12)
      n104 = call "AlliGator Get Tabulated Results Header (Decay Fit).vi"("Error In"=w79) -> ("Error Out"=w78:errorcluster, "Tabulated Results Header"=w98:string)  [unwired: 9 in]
      n105 = Build Array (concatenate)(w98, w99) -> (w97:string[])
      n106 = case shown="False" w96 {
        tunnel: w97 -> [w358 _]
        tunnel: [w357 w364] -> w95
        tunnel: w78 -> [w356 w364]
        tunnel: "Choose or enter file path for tabulated fits results:" ("prompt (Choose or enter file path)") -> [w355 _]
        tunnel: w93 -> [w354 _]
        frame False {
          n107 = case shown="True" w354 {
            tunnel: w358 -> [_ w363]
            tunnel: [w359 w362] -> w357
            tunnel: w356 -> [w359 w361]
            tunnel: w355 -> [_ w360]
            frame False {
            }
            frame True {
              n108 = Write to Text File(prompt (Choose or enter file path)=w360, text=w363, error in=w361) -> (error out=w362:errorcluster)  [unwired: 1 in, 2 out]
            }
          }
        }
        frame True {
        }
      }
    }
    n109 = in-place-dvr #1(w26) -> (→"AlliGator Internal Variables DVR":refnum<data-value>)  [unwired: 1 out]
  }
  n110 = call "High Resolution Timing.vi"("relative seconds (NaN)"=w14, "Error In"=w7) -> ("elapsed (relative) seconds"=w13:dbl, "Error Out"=w8:errorcluster)  [unwired: 15 in, 1 out]
  n111 = Array Size(array=w11) -> (size(s)=w10:i32)
  n112 = call "Concatenate String Array.vi"("Max Number of Elements (None: -1)"=8 ("Max Number of Elements (None: 1)"), "Separator (TAB)"=", ", "String Array"=w11) -> ("Formatted String"=w12:string)  [unwired: 8 in]
  n113 = call "Current Date & Time String (High Precision).vi"("Error In"=w8) -> ("on <Date> at <Time>"=w1:string)  [unwired: 7 in, 3 out]
  n114 = Format Into String(format string="All ROIs Decay Fit (%d):\n%scompleted %s\nCPU: %#g s\n", error in=w8, w10, w12, w1, w13) -> (resulting string=→"Message":string, error out=→"error out":errorcluster)  [unwired: 1 in]
